vi "HXG2_PlotScalesSaveFGV.vi"(6 "Plot Axis In":u32[](array[ring]) items=["1", "2", "3"], 7 "?":T1=enum."Plot Selection In", 8 "error in (no error)":errorcluster, 9 "Apply Scales":bool, 10 "Scales In":dbl[](array[numeric]), 11 "Plot Selection In":u16[](array[ring]) items=["none", "Liq In Avg", "Liq In 1", "Liq In 2", "Liq Out Avg", "Liq Out 1", "Liq Out 2", "Fltrd Mdot", "Liq Mdot", "Liq T° f/mtr", "Liq dP 0-25psi", "Liq Pin 0-100psi", "Air In Avg", "Air In 1", "Air In 2", "Air In 3", "Air In 4", "Air Out Avg", "Air Out 1", "Air Out 2", "Air Out 3", "Air Out 4", "Air Out 5", "Air Out 6", "Air Out 7", "Air Out 8", "CFM Nozzle", "CFM HX", "UUT 0-0.1inWC x100", "Chmb 0-5inWC x100", "Chmb 0-2.5inWC x100", "Liq Q (BTU/hr)", "Liq Q (W)", "Air Q (BTU/hr)", "Air Q (W)", "SH (°F)", "SH multiplier", "%Energy Bal", "Liq Re", "AF Ctl Out", "AC Ctl Out", "AH Ctl Out", "LF Ctl Out", "LC Ctl Out", "LH Ctl Out", "Box Btm In (9)", "Box Btm Out (10)", "Box Rt In (11)", "Box Rt Frt (12) ", "Box Top In(13)", "Box Top Out(14)", "Box Lt In (15)", "Box Lt Out (16)"]) -> (0 "error out":errorcluster, 1 "Apply Scales Out":bool, 2 "Scales Out":dbl[](array[numeric]), 3 "Plot Selection Out":u16[](array[numeric]), 4 "Plot Axis Out":u32[](array[numeric]))   [LabVIEW 2012]
uses:
  HXG2_GraphSelections.ctl
  <vilib>/Utility/file.llb/Read From Spreadsheet File (I64).vi
  <vilib>/Utility/file.llb/Read From Spreadsheet File (DBL).vi
  <vilib>/Utility/file.llb/Write To Spreadsheet File (DBL).vi
  <vilib>/Utility/file.llb/Write To Spreadsheet File (I64).vi
panel:
  out "Plot Axis In":path
  out "Graph Scales In":path
  out "Plot Selection In":path
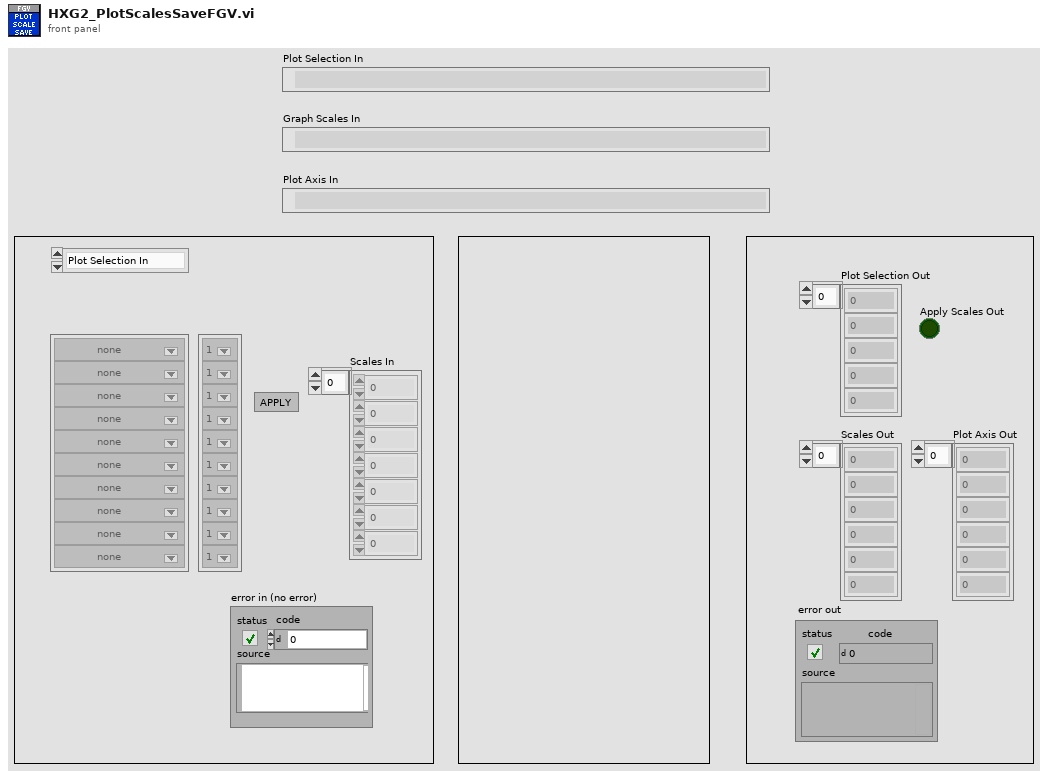
[diagram p1: front panel]
types:
  T1 = typedef "HXG2_GraphSelections.ctl" = enum16{"Load From File", "Plot Selection In", "Plot Axis In", "Graph Scales In", "Apply Scales", "Out"}
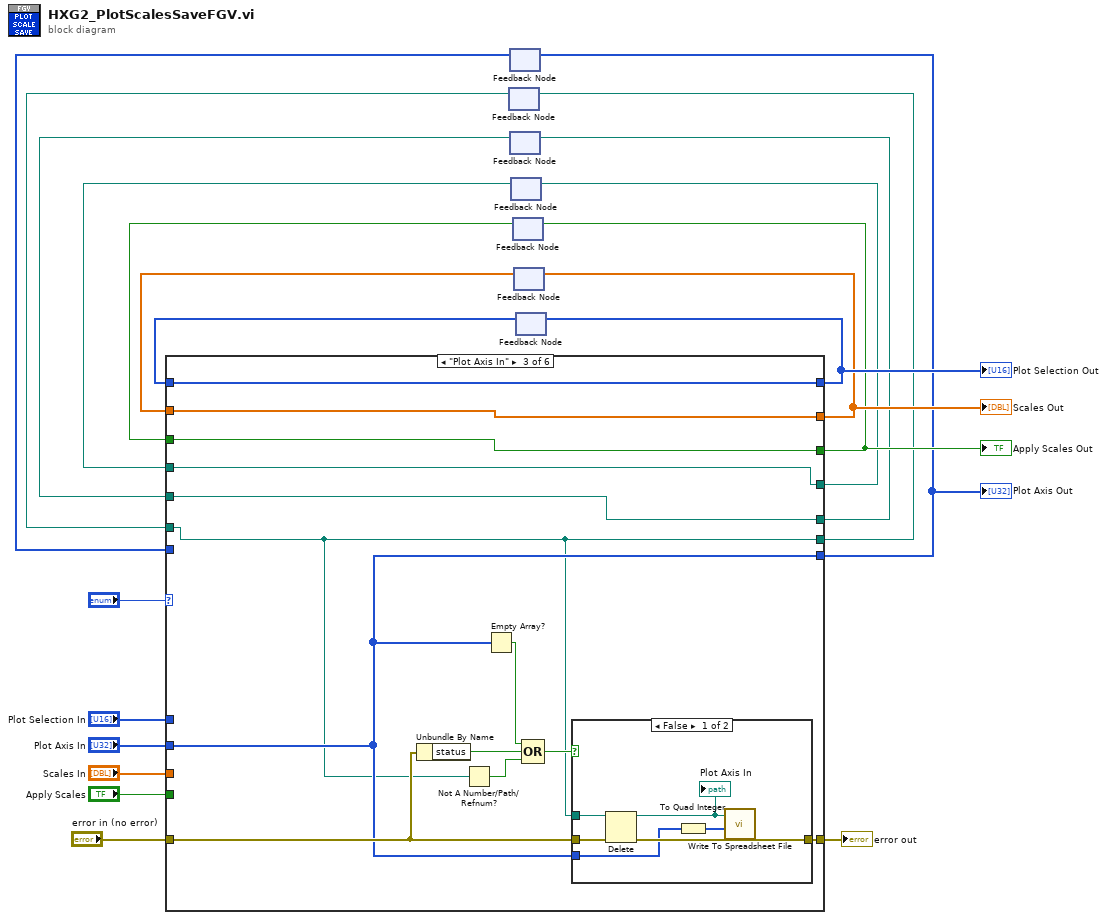
[diagram p0: block diagram]
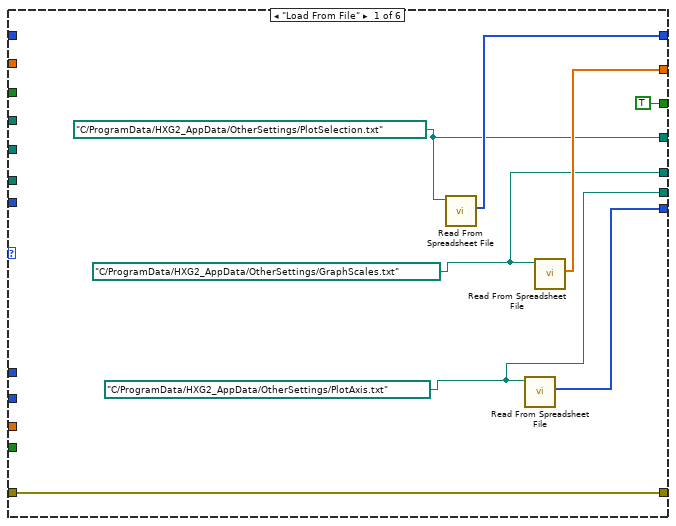
[diagram p2: hidden frame]
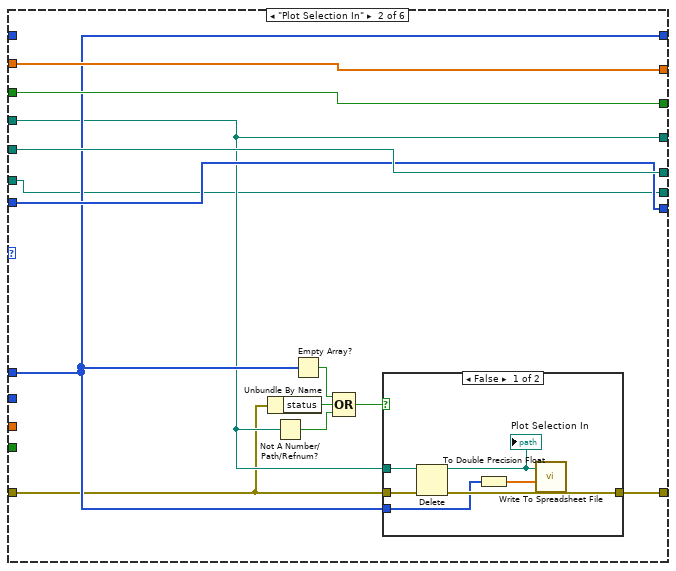
[diagram p3: hidden frame]
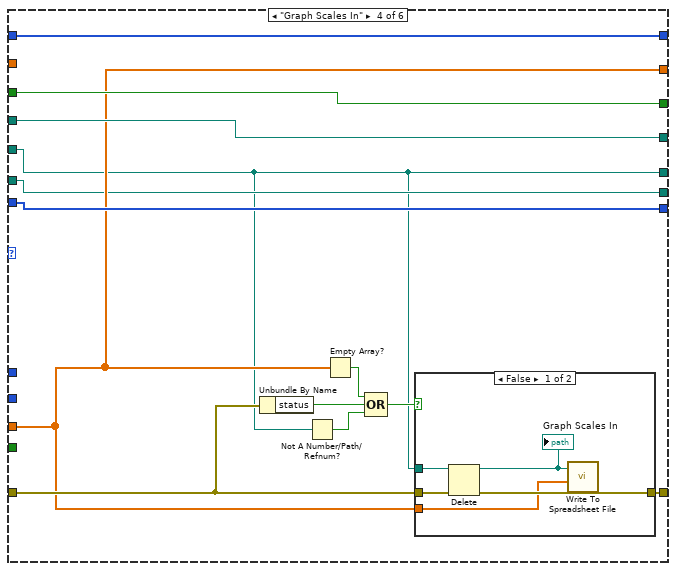
[diagram p6: hidden frame]
diagram:
  n1 = feedback #1() -> (w2:path)  [unwired: 1 in]
  n2 = feedback #2() -> (w4:i64[])  [unwired: 1 in]
  n3 = feedback #3() -> (w7:path)  [unwired: 1 in]
  n4 = feedback #4() -> (w9:path)  [unwired: 1 in]
  n5 = feedback #5() -> (w11:bool)  [unwired: 1 in]
  n6 = feedback #6() -> (w14:dbl[])  [unwired: 1 in]
  n7 = feedback #7() -> (w17:i64[])  [unwired: 1 in]
  n8 = case shown="\"Plot Axis In\"" "?" {
    tunnel: "error in (no error)" -> [w29 w31 w62 w82 w96 w104]
    tunnel: [w29 w42 w61 w81 w96 w104] -> w21
    tunnel: "Plot Selection In" -> [_ w33 _ _ _ _]
    tunnel: [w27 w33 w53 w72 w89 w103] -> w18
    tunnel: w17 -> [_ _ w53 w72 w89 w103]
    tunnel: "Scales In" -> [_ _ _ w73 _ _]
    tunnel: [w28 w37 w56 w73 w90 w102] -> w15
    tunnel: w14 -> [_ w37 w56 _ w90 w102]
    tunnel: "Apply Scales" -> [_ _ _ _ w92 _]
    tunnel: [TRUE ("Apply Scales") w36 w55 w76 w92 w101] -> w12
    tunnel: w11 -> [_ w36 w55 w76 _ w101]
    tunnel: [w26 w32 w50 w75 w95 w100] -> w10
    tunnel: w9 -> [_ w32 w50 w75 w95 w100]
    tunnel: [w25 w35 w54 w70 w94 w99] -> w8
    tunnel: w7 -> [_ w35 w54 w70 w94 w99]
    tunnel: "Plot Axis In" -> [_ _ w52 _ _ _]
    tunnel: [w24 w34 w52 w74 w93 w98] -> w5
    tunnel: w4 -> [_ w34 _ w74 w93 w98]
    tunnel: [w23 w30 w51 w71 w91 w97] -> w3
    tunnel: w2 -> [_ w30 w51 w71 w91 w97]
    frame "Load From File" {
      w23 = path "C:/ProgramData/HXG2_AppData/OtherSettings/PlotAxis.txt" ("File path")
      w25 = path "C:/ProgramData/HXG2_AppData/OtherSettings/GraphScales.txt" ("File path")
      w26 = path "C:/ProgramData/HXG2_AppData/OtherSettings/PlotSelection.txt" ("File path")
      n9 = call-poly <vilib>:"Read From Spreadsheet File.vi"("file path (dialog if empty)"=w26) -> ("first row"=w27:i64[])  [unwired: 6 in, 4 out]
      n10 = call-poly <vilib>:"Read From Spreadsheet File.vi"("file path (dialog if empty)"=w23) -> ("first row"=w24:i64[])  [unwired: 6 in, 4 out]
      n11 = call-poly <vilib>:"Read From Spreadsheet File.vi"("file path (dialog if empty)"=w25) -> ("first row"=w28:dbl[])  [unwired: 6 in, 4 out]
    }
    frame "Plot Selection In" {
      n12 = Unbundle By Name(w31) -> ("status"=w41:bool)
      n13 = Not A Number/Path/Refnum?(number/path/refnum=w32) -> (NaN/Path/Refnum?=w40:bool)
      n14 = Empty Array?(array=w33) -> (empty?=w39:bool)
      n15 = Compound Arithmetic op=OR(w39, w41, w40) -> (w38:bool)
      n16 = case shown="False" w38 {
        tunnel: w33 -> [w45 _]
        tunnel: w31 -> [w47 w49]
        tunnel: [w46 w49] -> w42
        tunnel: w32 -> [w44 _]
        frame False {
          n17 = Delete(path (use dialog)=w44, error in=w47) -> (deleted path=w48:path, error out=w46:errorcluster)  [unwired: 4 out]
          "Plot Selection In" <- w48
          n18 = To Double Precision Float(number=w45) -> (double precision float=w43:dbl[])
          n19 = call-poly <vilib>:"Write To Spreadsheet File.vi"("1D data"=w43, "file path (dialog if empty)"=w48) -> ()  [unwired: 4 in, 3 out]
        }
        frame True {
        }
      }
    }
    frame "Plot Axis In" {
      n20 = Unbundle By Name(w62) -> ("status"=w60:bool)
      n21 = Not A Number/Path/Refnum?(number/path/refnum=w51) -> (NaN/Path/Refnum?=w59:bool)
      n22 = Empty Array?(array=w52) -> (empty?=w58:bool)
      n23 = Compound Arithmetic op=OR(w58, w60, w59) -> (w57:bool)
      n24 = case shown="False" w57 {
        tunnel: w52 -> [w64 _]
        tunnel: w62 -> [w67 w69]
        tunnel: [w66 w69] -> w61
        tunnel: w51 -> [w65 _]
        frame False {
          n25 = Delete(path (use dialog)=w65, error in=w67) -> (deleted path=w68:path, error out=w66:errorcluster)  [unwired: 4 out]
          "Plot Axis In" <- w68
          n26 = To Quad Integer(1:w64) -> (0:w63:i64[])
          n27 = call-poly <vilib>:"Write To Spreadsheet File.vi"("1D data"=w63, "file path (dialog if empty)"=w68) -> ()  [unwired: 4 in, 3 out]
        }
        frame True {
        }
      }
    }
    frame "Graph Scales In" {
      n28 = Unbundle By Name(w82) -> ("status"=w80:bool)
      n29 = Not A Number/Path/Refnum?(number/path/refnum=w70) -> (NaN/Path/Refnum?=w79:bool)
      n30 = Empty Array?(array=w73) -> (empty?=w78:bool)
      n31 = Compound Arithmetic op=OR(w78, w80, w79) -> (w77:bool)
      n32 = case shown="False" w77 {
        tunnel: w73 -> [w84 _]
        tunnel: w82 -> [w86 w88]
        tunnel: [w85 w88] -> w81
        tunnel: w70 -> [w83 _]
        frame False {
          n33 = Delete(path (use dialog)=w83, error in=w86) -> (deleted path=w87:path, error out=w85:errorcluster)  [unwired: 4 out]
          "Graph Scales In" <- w87
          n34 = call-poly <vilib>:"Write To Spreadsheet File.vi"("1D data"=w84, "file path (dialog if empty)"=w87) -> ()  [unwired: 4 in, 3 out]
        }
        frame True {
        }
      }
    }
    frame "Apply Scales" {
    }
    frame "Out" {
    }
  }
  "error out" <- w21
  "Plot Selection Out" <- w18
  "Scales Out" <- w15
  "Apply Scales Out" <- w12
  "Plot Axis Out" <- w5
  n35 = feedback-in #1(w3) -> ()
  n36 = feedback-in #2(w5) -> ()
  n37 = feedback-in #3(w8) -> ()
  n38 = feedback-in #4(w10) -> ()
  n39 = feedback-in #5(w12) -> ()
  n40 = feedback-in #6(w15) -> ()
  n41 = feedback-in #7(w18) -> ()
